vi "Demo_SaveImageToFile.vi"() -> ()   [LabVIEW 2024]
doc: "Save image in any formats supported by QuickTime.\nUse QT_Info.vi to learn about QT supported formats.\n\n© Ch. Salzmann, 1994-2003"
uses:
  <userlib>/ImageProcessing/QTLIB_2595_LV86/QT_Private.ctl
  <userlib>/ImageProcessing/QTLIB_2595_LV86/QT_File.ctl
  <userlib>/ImageProcessing/QTLIB_2595_LV86/QT_Compression.ctl
panel:
  in  "Format":u16(ring) items=["BMP", "JPEG", "MacPaint", "Photoshop", "PNG", "PICT", "QuickTime", "SG", "Targa", "TIFF"]
  in  "Compression":i32(slide) scale=0.0..1023.0 scale format="%.0x"
  out "Image Source":picture
  out "error out":errorcluster
  in  "Image path":path=path "/Chris/new Chris/Projects/FAT-CIN prj/FatCIN/Test_Prg/img.jpg"
  # "Save image in any formats\nsupported by QuickTime\n© Ch. Salzmann, 1994-2005"
  # "Min"
  # "Low"
  # "Normal"
  # "Hight"
  # "Max"
  # "Loss less"
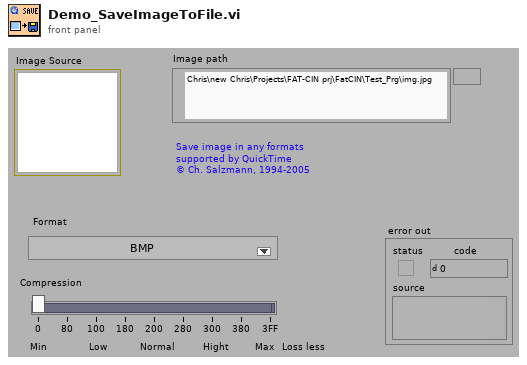
[diagram p1: front panel]
types:
  T1 = typedef "QT_Compression.ctl" = cluster{"Compression":i32, "Format":i32, "Codec":i32, "Comp. Quality":i32, "Key Frame":i32, "Dialogs":u32}
  T2 = typedef "QT_File.ctl" = cluster{"Paths":string[], "Options":i32, "Dialogs":u32, "Reserved":i32}
  T3 = typedef "QT_Private.ctl" = cluster{"reserved 1":i32, "reserved 2":i32, "reserved 3":i32, "reserved 4":i32}
  T4 = typedef "QT_Image.ctl" = cluster{"Width":i32, "Height":i32, "Depth":i32, "data":u8[], "Compressed data":u8[], "Color table":u32[], "Duration":i32, "Options":i32, "Timestamp":i32, "ID":i32, "Reserved":i32, "Dialogs":u32}
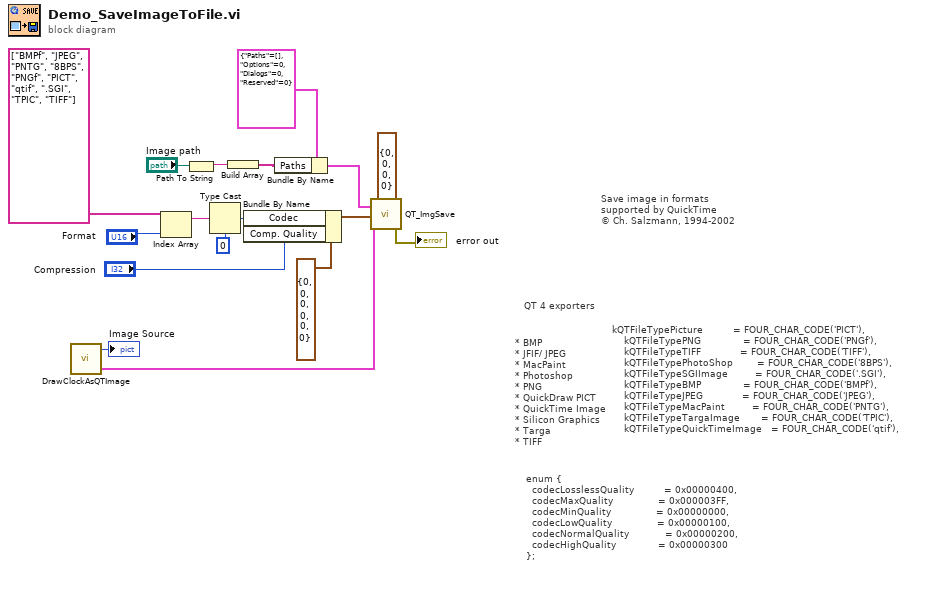
[diagram p0: block diagram]
diagram:
  # "QT 4 exporters"
  # "* BMP\n*\tJFIF/ JPEG \n*\tMacPaint\n*\tPhotoshop \n*\tPNG\n*\tQuickDraw PICT \n*\tQuickTime Image \n*\tSilicon Graphics\n*\tTarga\n*\tTIFF"
  # "kQTFileTypePicture          = FOUR_CHAR_CODE('PICT'),\n    kQTFileTypePNG              = FOUR_CHAR_CODE('PNGf'),\n    kQTFileTypeTIFF             = FOUR_CHAR_CODE('TIFF'),\n    kQTFileTypePhotoShop        = FOUR_CHAR_CODE('8BPS'),\n    kQTFileTypeSGIImage         = FOUR_CHAR_CODE('.SGI'),\n    kQTFileTypeBMP              = FOUR_CHAR_CODE('BMPf'),\n    kQTFileTypeJPEG             = FOUR_CHAR_CODE('JPEG'),\n    kQTFileTypeMacPaint         = FOUR_CHAR_CODE('PNTG'),\n    kQTFileTypeTargaImage       = FOUR_CHAR_CODE('TPIC'),\n    kQTFileTypeQuickTimeImage   = FOUR_CHAR_CODE('qtif'),"
  # "enum {\n  codecLosslessQuality          = 0x00000400,\n  codecMaxQuality               = 0x000003FF,\n  codecMinQuality               = 0x00000000,\n  codecLowQuality               = 0x00000100,\n  codecNormalQuality            = 0x00000200,\n  codecHighQuality              = 0x00000300\n};"
  # "Save image in formats\nsupported by QuickTime\n© Ch. Salzmann, 1994-2002"
  n1 = call <userlib>:"DrawClockAsQTImage.vi"() -> ("Picture"=→"Image Source":picture, "Image Out (24 bits)"=w9:T4)  [unwired: 2 in, 16 out]
  n2 = Index Array(array=string[] ["BMPf", "JPEG", "PNTG", "8BPS", "PNGf", "PICT", "qtif", ".SGI", "TPIC", "TIFF"], index="Format") -> (element=w4:string)
  n3 = Path To String(path="Image path") -> (string=w16:string)
  n4 = Type Cast(type=0 ("Format"), x=w4) -> (*(type *) &x=w2:i32)
  n5 = Build Array(w16) -> (w1:string[])
  n6 = Bundle By Name(cluster=T1 {"Compression"=0, "Format"=0, "Codec"=0, "Comp. Quality"=0, "Key Frame"=0, "Dialogs"=0} ("Compression Settings"), "Codec"=w2, "Comp. Quality"="Compression") -> (w13:T1)
  n7 = Bundle By Name(cluster=T2 {"Paths"=[], "Options"=0, "Dialogs"=0, "Reserved"=0} ("File Settings"), "Paths"=w1) -> (w10:T2)
  n8 = call <userlib>:"QT_ImgSave.vi"("File Settings"=w10, "Image In"=w9, "Compression Settings"=w13, "Private"=T3 {"reserved 1"=0, "reserved 2"=0, "reserved 3"=0, "reserved 4"=0}) -> ("error out"=→"error out":errorcluster)  [unwired: 5 in, 10 out]
